vi "test-single-jointed-arm-sim.vi"(8 "error in (no error)":errorcluster) -> (0 "error out":errorcluster, 3 "Test Passed":bool)   [LabVIEW 2019]
uses:
  <vilib>/Rock Robotics/WPI/ThirdParty/JAS_Junk/TrajLib/Trajectory_Library.lvlib
  <vilib>/Rock Robotics/WPI/ThirdParty/JAS_Junk/TrajLib/DCMotor_GetVex775Pro.vi
  <vilib>/Analysis/Matrix/Datatypes/RealMatrix.ctl
  <vilib>/Analysis/Matrix/NI_Matrix.lvlib
  <vilib>/Rock Robotics/WPI/ThirdParty/JAS_Junk/TrajLib/TypeDef/LINEAR_SYSTEM.ctl
  <vilib>/Rock Robotics/WPI/ThirdParty/JAS_Junk/TrajLib/TypeDef/DCMOTOR.CTL
  <vilib>/Rock Robotics/WPI/ThirdParty/JAS_Junk/TrajLib/TypeDef/LINEAR_SYSTEM_SIM.ctl
  <vilib>/Rock Robotics/WPI/ThirdParty/JAS_Junk/TrajLib/TypeDef/SINGLE_JOINT_ARM_SIM.ctl
panel:
  in  "Tab Control":enum32{"Operation", "Motor", "Arm Sim"}(tab)
  out "Velocity RAD/SEC":cluster{"Voltage":dbl}(graph)
  out "PV Chart":cluster{dbl}(graph)
  out "Position RAD":dbl
  in  "Input_Voltage":dbl format="%#_13g"
  out "Arm Motor":T1 {"Jr_KgM2" format="%13.5p"; "L_H" format="%13.5p"; "Kt_NMPerAmp" format="%13.5p"; "KvINV_RadPerSecPerVolt" format="%13.5p"; "R_Ohms" format="%13.5p"; "FreeSpeed_RadPerSec" format="%13.5p"; "FreeCurrent_Amps" format="%13.5p"; "StallCurrent_Amps" format="%13.5p"; "StallTorque_NM" format="%13.5p"; "nominalVoltage_Volts" format="%13.5p"}
  out "Arm Simulaation":T2 {"GearBox"."Jr_KgM2" format="%13.5p"; "GearBox"."L_H" format="%13.5p"; "GearBox"."Kt_NMPerAmp" format="%13.5p"; "GearBox"."KvINV_RadPerSecPerVolt" format="%13.5p"; "GearBox"."R_Ohms" format="%13.5p"; "GearBox"."FreeSpeed_RadPerSec" format="%13.5p"; "GearBox"."FreeCurrent_Amps" format="%13.5p"; "GearBox"."StallCurrent_Amps" format="%13.5p"; "GearBox"."StallTorque_NM" format="%13.5p"; "GearBox"."nominalVoltage_Volts" format="%13.5p"}
  # "<States, 1>"
  # "<Outputs, 1>"
  # "<Inputs, 1>"
  # "<Outputs, 1>"
  # "<States,States>"
  # "<States,Inputs>"
  # "<Outputs,States>"
  # "<Outputs,Inputs>"
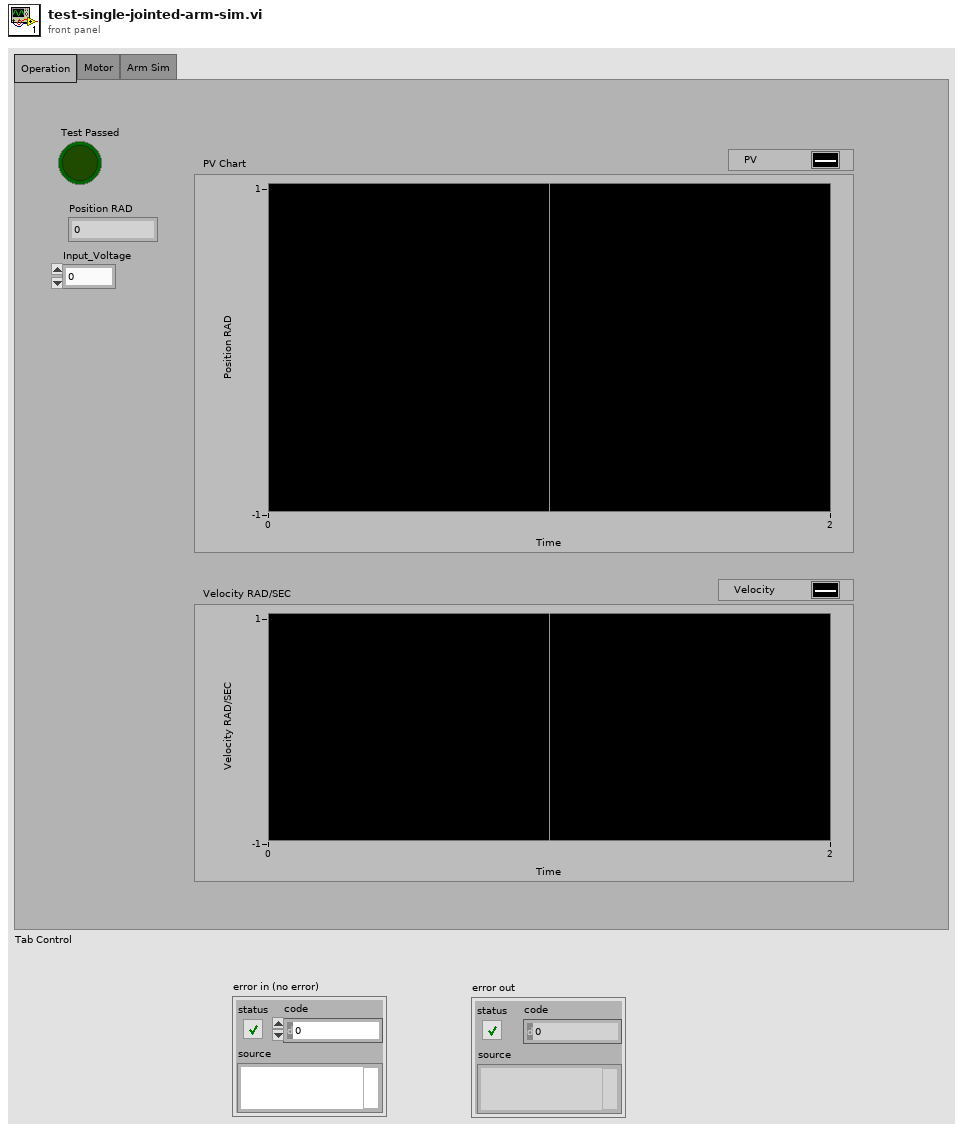
[diagram p1: front panel]
types:
  T1 = typedef "Trajectory_Library.lvlib/DCMOTOR.CTL" = cluster{"nominalVoltage_Volts":dbl, "StallTorque_NM":dbl, "StallCurrent_Amps":dbl, "FreeCurrent_Amps":dbl, "FreeSpeed_RadPerSec":dbl, "R_Ohms":dbl, "KvINV_RadPerSecPerVolt":dbl, "Kt_NMPerAmp":dbl, "L_H":dbl, "Jr_KgM2":dbl}
  T2 = typedef "Trajectory_Library.lvlib/SINGLE_JOINT_ARM_SIM.ctl" = cluster{"Arm_LinearSystem":T3, "GearBox":T1, "Gearing":dbl, "R_ArmLength_M":dbl, "MinAngle_Rad":dbl, "MaxAngle_Rad":dbl, "SimulateGravity":bool}
  T3 = typedef "Trajectory_Library.lvlib/LINEAR_SYSTEM_SIM.ctl" = cluster{"m_Plant":T4, "m_X":T5, "m_Y":T5, "m_U":T5, "MeasureStdDev":T5}
  T4 = typedef "Trajectory_Library.lvlib/LINEAR_SYSTEM.ctl" = cluster{"m_A":T5, "m_B":T5, "m_C":T5, "m_D":T5, "States":i32, "Inputs":i32, "Outputs":i32}
  T5 = typedef "NI_Matrix.lvlib/RealMatrix.ctl" = dbl[][]
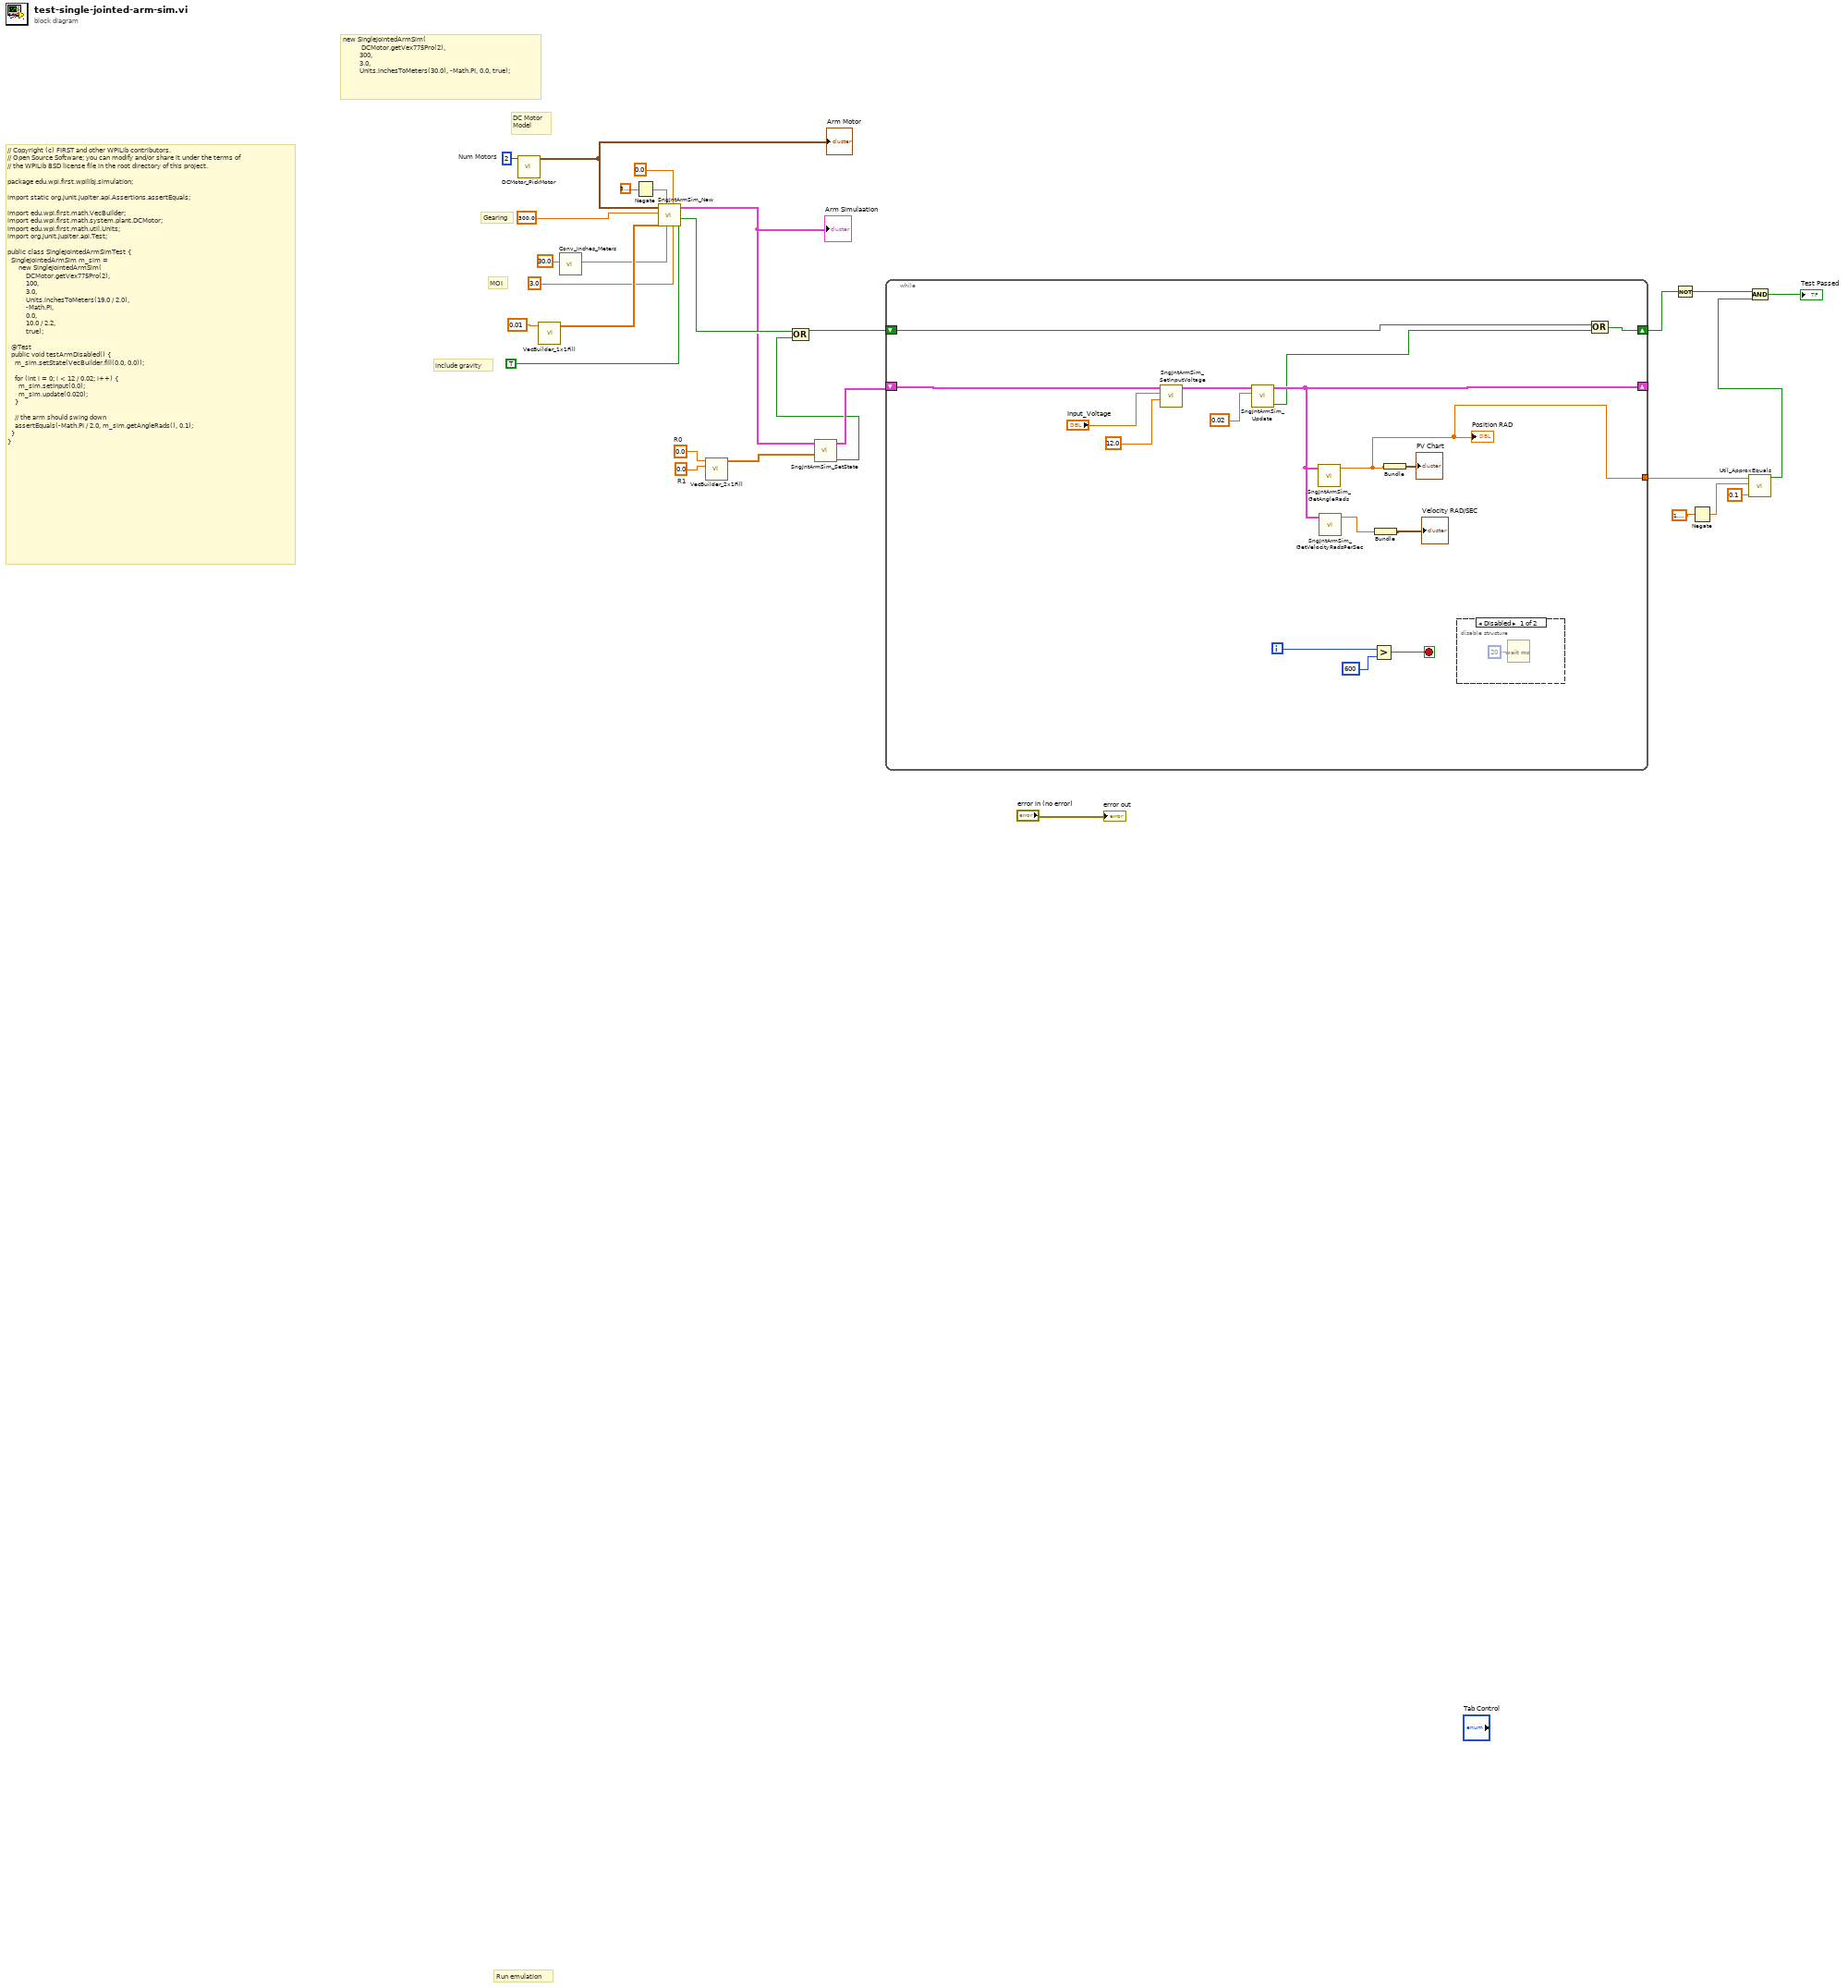
[diagram p0: block diagram]
diagram:
  w3 = 2  # Num Motors
  w9 = 0.0  # R1
  w8 = 0.0  # R0
  # "DC Motor\nModel"
  # "include gravity"
  # "MOI"
  # "Gearing"
  # "// Copyright (c) FIRST and other WPILib contributors.\n// Open Source Software; you can modify and/or share it under the terms of\n// the WPILib BSD license file in the root directory of this project.\n\npackage edu.wpi.first.wpilibj.simulation;\n\nimport static org.junit.jupiter.api.Assertions.assertEquals;\n\nimport edu.wpi.first.math.VecBuilder;\nimport edu.wpi.first.math.system.plant.DCMotor;\nimport edu.wpi.first.math.util.Units;\nimport org.junit.jupiter.api.Test;\n\npublic class SingleJointedArmSimTest {\n  SingleJointedArmSim m_sim =\n      new SingleJointedArmSim(\n          DCMotor.getVex775Pro(2),\n          100,\n          3.0,\n          Units.inchesToMeters(19.0 / 2.0),\n          -Math.PI,\n          0.0,\n          10.0 / 2.2,\n          true);\n\n  @Test\n  public void testArmDisabled() {\n    m_sim.setState(VecBuilder.fill(0.0, 0.0));\n\n    for (int i = 0; i < 12 / 0.02; i++) {\n      m_sim.setInput(0.0);\n      m_sim.update(0.020);\n    }\n\n    // the arm should swing down\n    assertEquals(-Math.PI / 2.0, m_sim.getAngleRads(), 0.1);\n  }\n}"
  # "new SingleJointedArmSim(\n          DCMotor.getVex775Pro(2), \n         300, \n         3.0, \n         Units.inchesToMeters(30.0), -Math.PI, 0.0, true);"
  # "Run emulation"
  n1 = call-poly <vilib>:"DCMotor_PickMotor.vi"("Num Motors"=w3) -> ("DCMOTOR"=w2:T1)  [unwired: 10 in]
  "Arm Motor" <- w2
  n2 = call <vilib>:"VecBuilder_1x1Fill.vi"("R0_C0"=0.01) -> ("output matrix"=w25:T5)  [unwired: 10 in]
  n3 = call <vilib>:"Conv_Inches_Meters.vi"("INCH"=30.0) -> ("Meters"=w17:dbl)  [unwired: 10 in]
  n4 = Negate(x=3.141592653589793) -> (-x=w15:dbl)
  n5 = call <vilib>:"SngJntArmSim_New.vi"("SimulateGravity"=TRUE, "jKgMetersSquared"=3.0, "MaxAngle_Rad"=0.0 ("MaxHeight_Meters"), "ArmLength_Meters"=w17, "MinAngle_Rad"=w15, "MeasurementStdDev"=w25, "Gearing"=300.0, "GearBox"=w2) -> ("Error"=w24:bool, "SingleJointArmSim"=w12:T2)  [unwired: 2 in]
  "Arm Simulaation" <- w12
  n6 = call <vilib>:"VecBuilder_2x1Fill.vi"("R1"=w9, "R0"=w8) -> ("output matrix"=w7:T5)  [unwired: 9 in]
  n7 = call <vilib>:"SngJntArmSim_SetState.vi"("System State"=w7, "in ArmSim"=w12) -> ("Size Coerced"=w10:bool, "out ArmSim"=w11:T2)  [unwired: 8 in]
  n8 = Compound Arithmetic op=OR(w24, w10) -> (w28:bool)
  n9 = while {
    shift-right: [w33] -> _
    shift-left: w11 -> [w35]
    shift-right: [w41] -> w20
    shift-left: w28 -> [w42]
    tunnel: [w31] -> w13
    i -> [w45]
    stop <- w43 stop-if-true
    n10 = call <vilib>:"SngJntArmSim_SetInputVoltage.vi"("Battery_Volts"=12.0, "Input_Voltage"="Input_Voltage", "in SingleJointArmSim"=w35) -> ("out SingleJointArmSim"=w40:T2)  [unwired: 8 in]
    n11 = call <vilib>:"SngJntArmSim_Update.vi"("dT_Seconds"=0.02, "in SingleJointArmSim"=w40) -> ("Error"=w30:bool, "out SingleJointArmSim"=w33:T2)  [unwired: 8 in]
    n12 = call <vilib>:"SngJntArmSim_GetAngleRads.vi"("SingleJointArmSim"=w33) -> ("ArmAngle_Rad"=w31:dbl)  [unwired: 10 in]
    "Position RAD" <- w31
    n13 = call <vilib>:"SngJntArmSim_GetVelocityRadsPerSec.vi"("singleJointArmSim"=w33) -> ("Velocity_RadsPerSec"=w32:dbl)  [unwired: 10 in]
    n14 = Greater?(x=w45, y=600) -> (0:w43:bool)
    n15 = Bundle("Velocity_RadsPerSec"=w32) -> (→"Velocity RAD/SEC":cluster{"Velocity_RadsPerSec":dbl})  [unwired: 1 in]
    n16 = Bundle("ArmAngle_Rad"=w31) -> (→"PV Chart":cluster{"ArmAngle_Rad":dbl})  [unwired: 1 in]
    n17 = disable-structure shown="Disabled" {
      frame Disabled {
        n18 = Wait (ms)(milliseconds to wait=u32 20) -> ()  [unwired: 1 out]
      }
      frame Enabled {
      }
    }
    n19 = Compound Arithmetic op=OR(w42, w30) -> (w41:bool)
  }
  n20 = Not(x=w20) -> (.not. x?=w19:bool)
  n21 = Negate(x=1.5707963267948966) -> (-x=w5:dbl)
  n22 = call <vilib>:"Util_ApproxEquals.vi"("Tolerance"=0.1, "Value 2"=w5, "Value 1"=w13) -> ("ApproxEquals"=w21:bool)  [unwired: 8 in]
  n23 = Compound Arithmetic op=AND(w19, w21) -> (→"Test Passed":bool)
  "error out" <- "error in (no error)"
